vi "顶层容器-有线上位机.vi"() -> ()   [LabVIEW 2017]
panel:
  out "查-刷新设备表 按钮":refnum<vi>
  out "查-查询今日 按钮":refnum<vi>
  out "累积查询窗口VI-引用":refnum<vi>
  out "管-更新列表状态？":refnum<vi>
  out "管-停止信号（枚举）":refnum<vi>
  out "管-监测窗口 按钮":refnum<vi>
  in  "监-外部停止信号":refnum<vi>
  out "管理窗口VI-引用":refnum<vi>
  out "管-监测窗口VI-控件引用":refnum<vi>
  in  "管理模式":bool
  in  "监测模式":bool
  in  "累积查询":bool
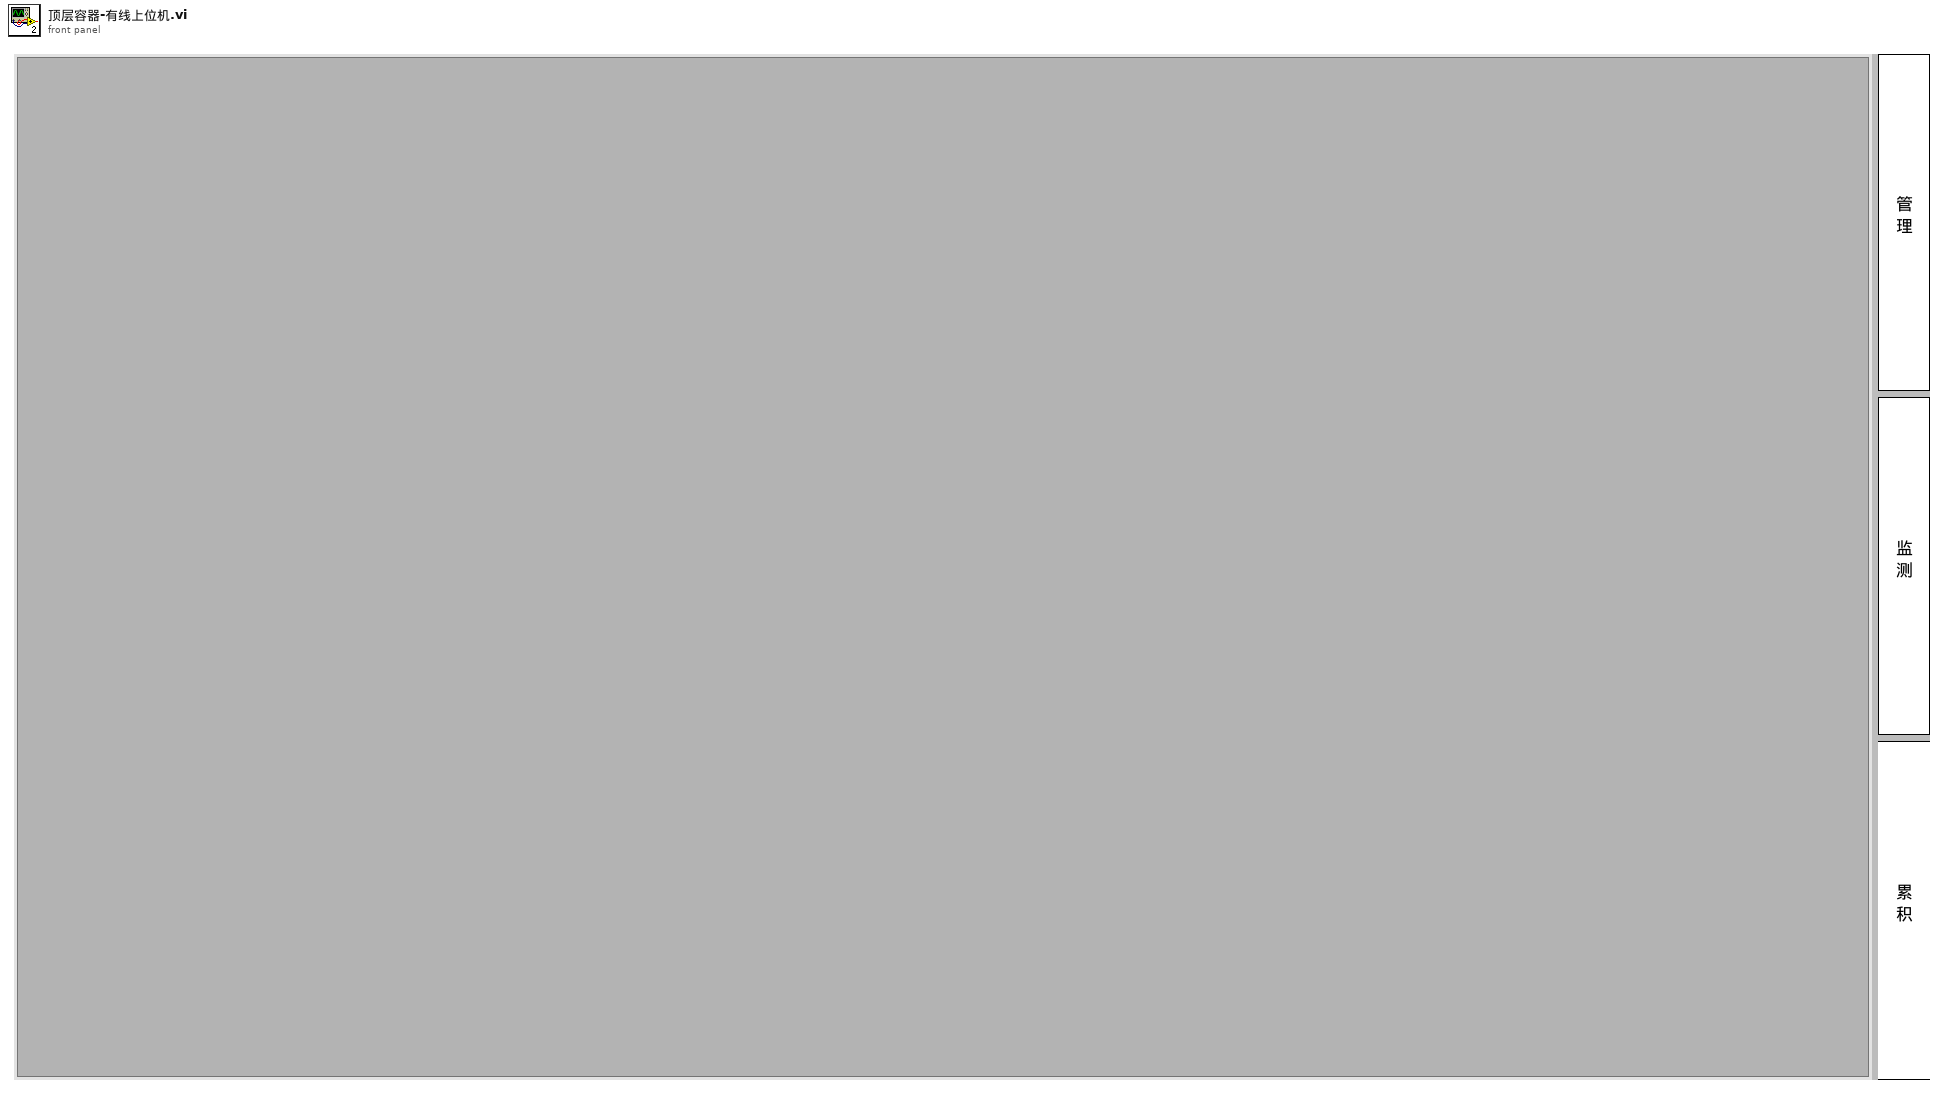
[diagram p1: front panel]
types:
  T1 = enum8{"Enabled", "Disabled", "Disabled and Grayed Out"}
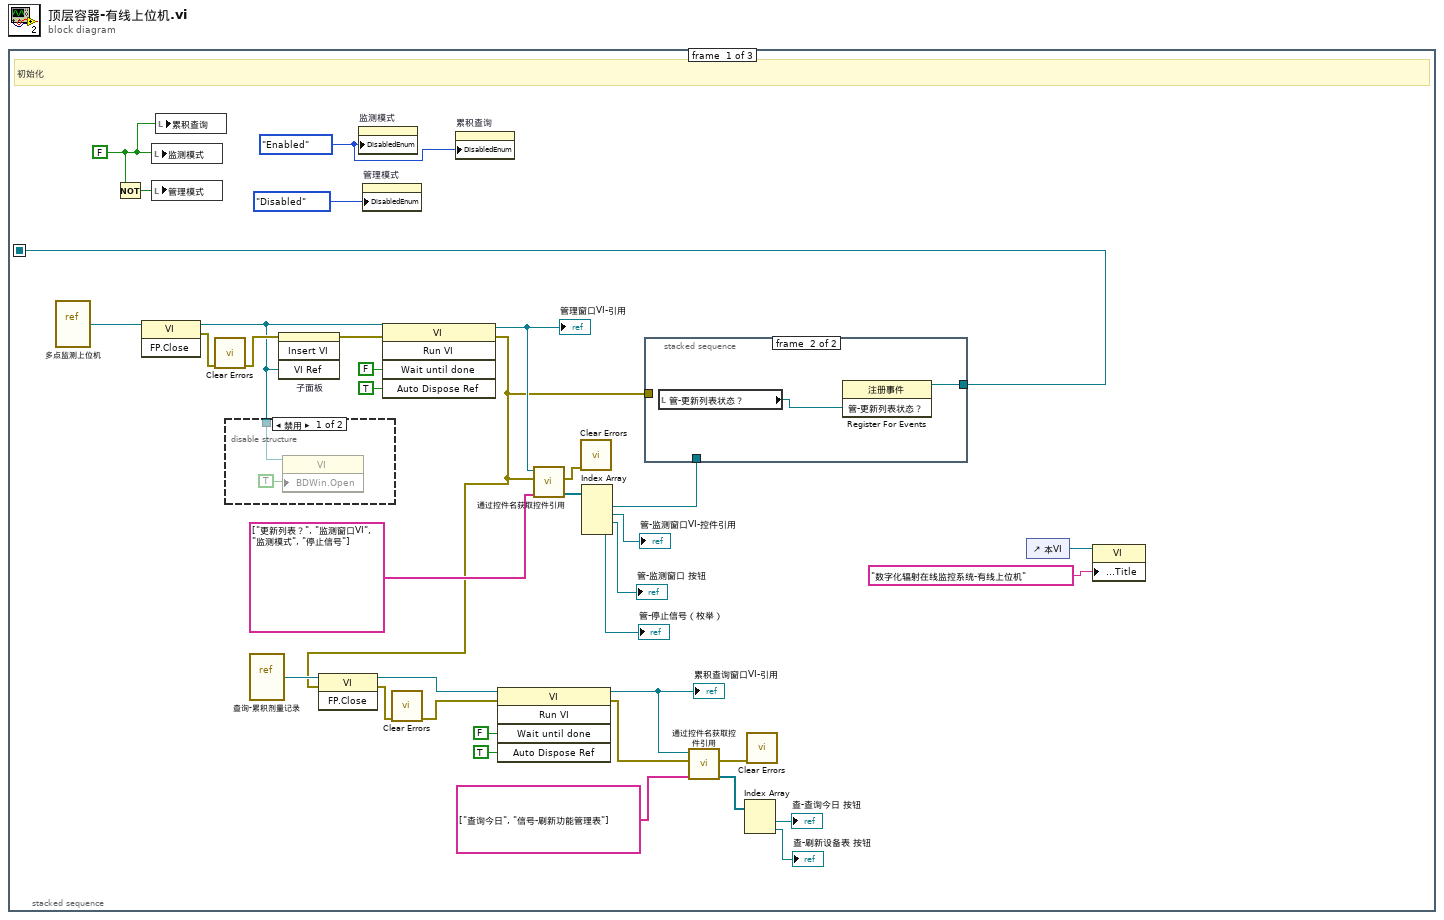
[diagram p0: block diagram]
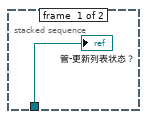
[diagram p3: hidden frame]
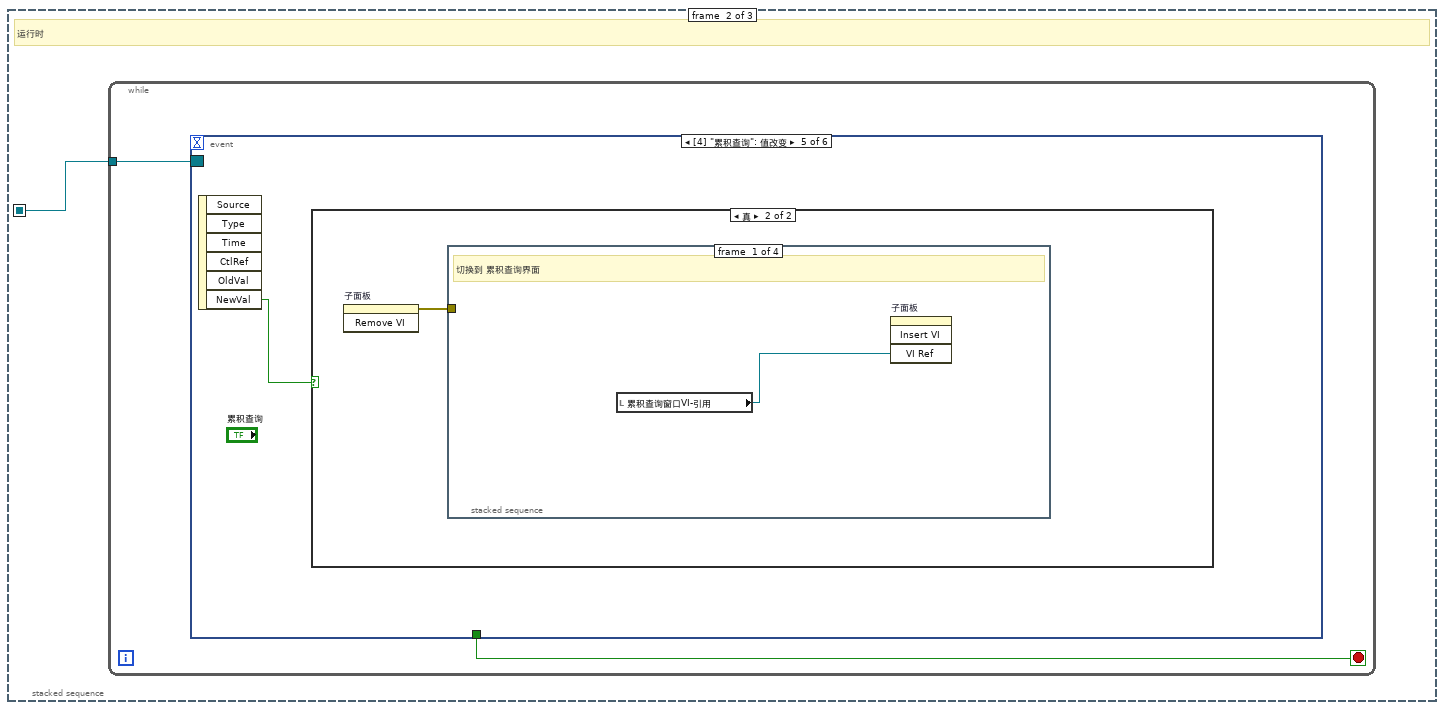
[diagram p4: hidden frame]
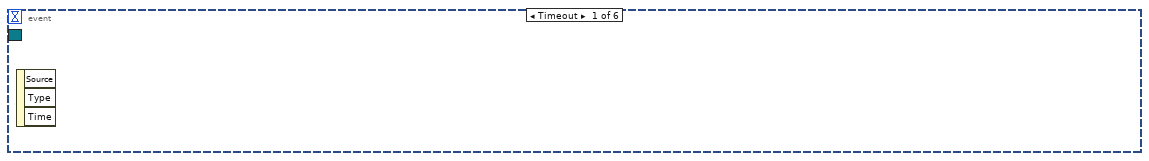
[diagram p5: hidden frame]
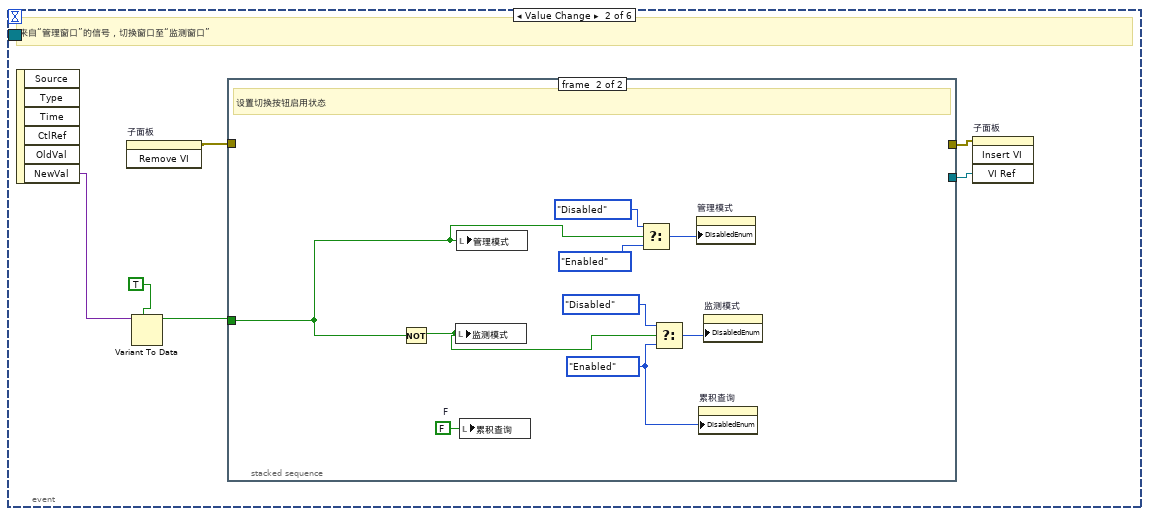
[diagram p6: hidden frame]
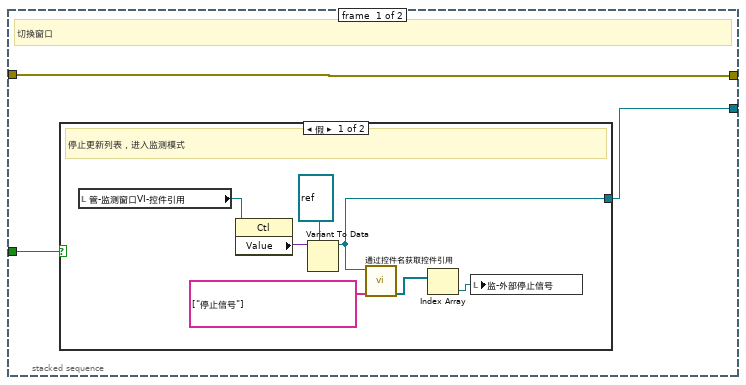
[diagram p7: hidden frame]
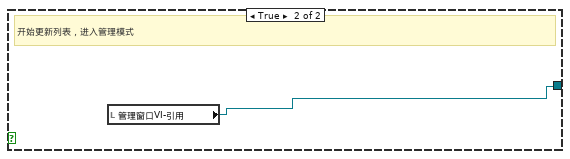
[diagram p8: hidden frame]
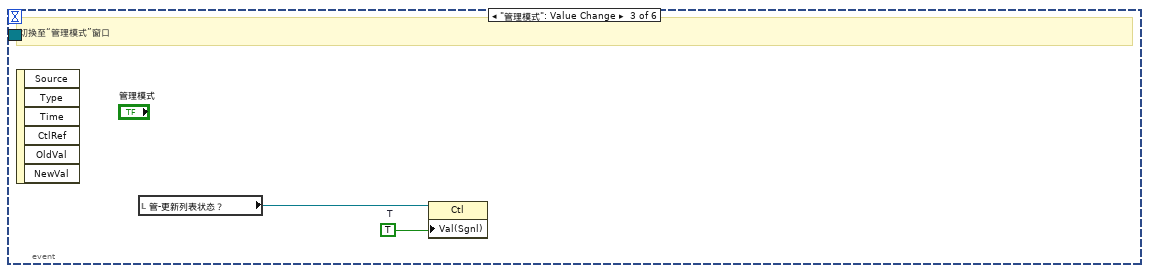
[diagram p9: hidden frame]
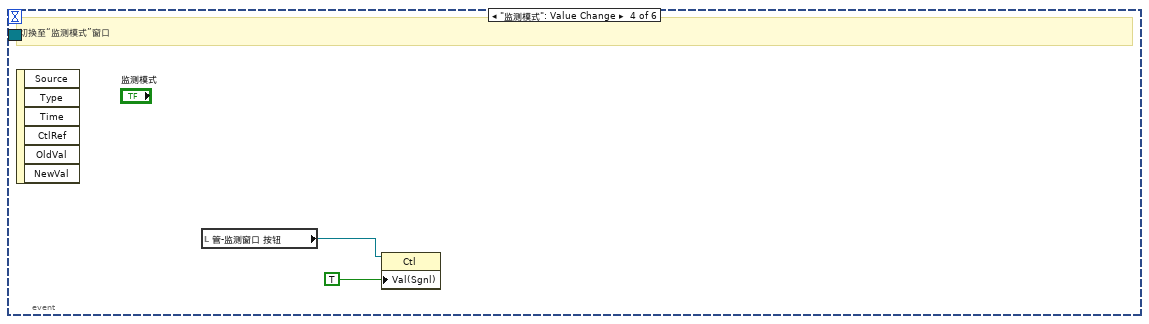
[diagram p10: hidden frame]
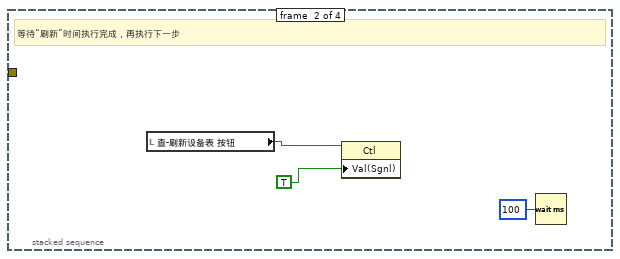
[diagram p12: hidden frame]
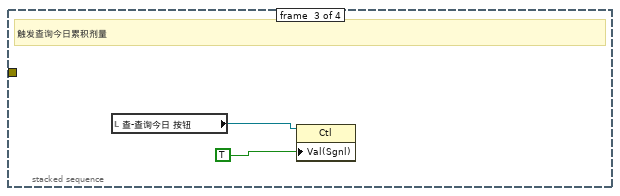
[diagram p13: hidden frame]
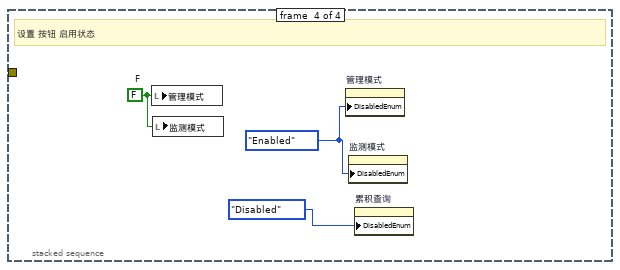
[diagram p14: hidden frame]
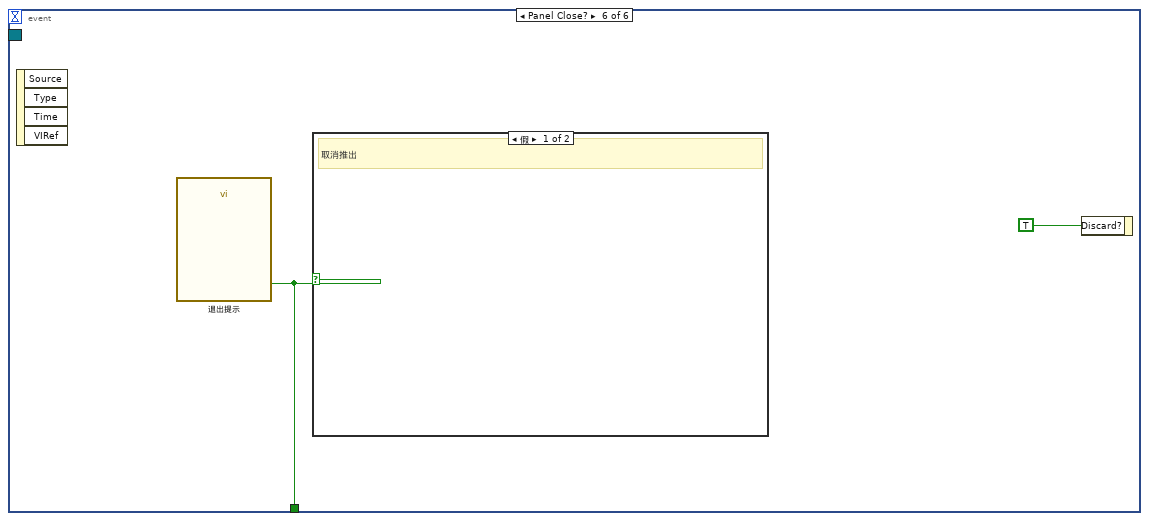
[diagram p15: hidden frame]
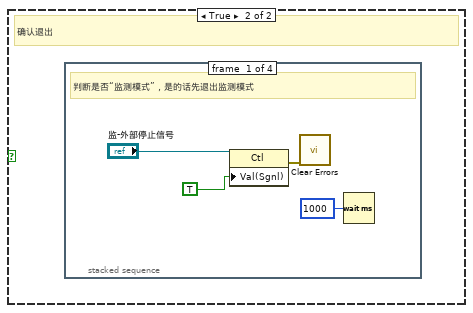
[diagram p16: hidden frame]
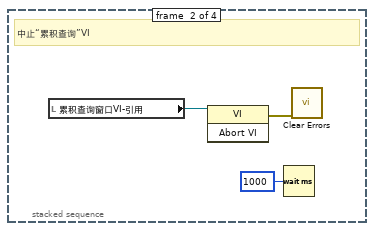
[diagram p17: hidden frame]
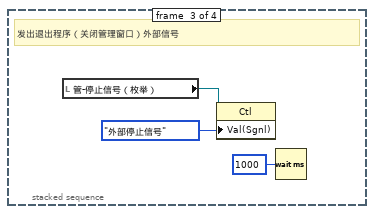
[diagram p18: hidden frame]
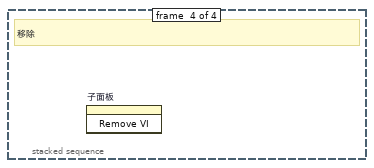
[diagram p19: hidden frame]
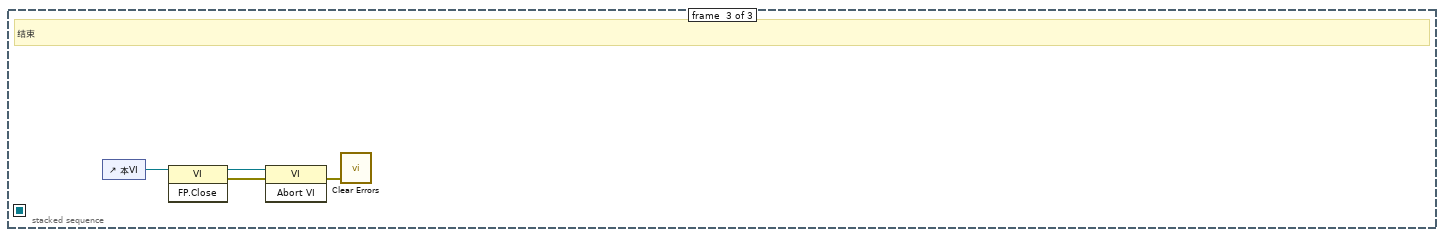
[diagram p20: hidden frame]
diagram:
  n1 = stacked-sequence {
    seq-local: [w31 _ _] -> [_ w42 _]
    frame #0 {
      w5 = T1."Enabled" ("禁用")
      w4 = FALSE ("监测模式")
      # "初始化"
      n2 = vi-ref "多点监测上位机.vi"() -> (w24:refnum<vi>)
      n3 = Not(x=w4) -> (.not. x?=w6:bool)
      n4 = invoke class="VI" method="FP.Close"(reference=w24) -> (reference out=w20:refnum<vi>, error out=w22:errorcluster)  [unwired: 2 in, 1 out]
      n5 = local write "监测模式"(w4) -> ()
      n6 = local write "管理模式"(w6) -> ()
      n7 = local write "累积查询"(w4) -> ()
      n8 = call <vilib>:"Clear Errors.vi"("error in (no error)"=w22) -> ("error out"=w21:errorcluster)  [unwired: 5 in, 1 out]
      n9 = disable-structure shown="禁用" {
        disable-tunnel: w20 -> [w38 _]
        frame Disabled {
          n10 = property class="VI"(reference=w38, "BDWin.Open"=TRUE ("程序框图窗口:打开")) -> ()  [unwired: 1 in, 2 out]
        }
        frame Enabled {
        }
      }
      n11 = vi-ref "查询-累积剂量记录.vi"() -> (w16:refnum<vi>)
      n12 = invoke on="子面板" class="子面板" method="Insert VI"(error in=w21, "VI Ref"=w20) -> (error out=w19:errorcluster)  [unwired: 2 in, 3 out]
      n13 = property on="监测模式" class="Bool (严格)"("DisabledEnum"=w5) -> ()  [unwired: 2 in, 2 out]
      n14 = property on="管理模式" class="Bool (严格)"("DisabledEnum"=T1."Disabled" ("禁用")) -> ()  [unwired: 2 in, 2 out]
      n15 = invoke class="VI" method="Run VI"(reference=w20, error in=w19, "Wait until done"=FALSE ("结束前等待"), "Auto Dispose Ref"=TRUE ("自动销毁引用")) -> (reference out=w32:refnum<vi>, error out=w1:errorcluster)  [unwired: 1 in, 3 out]
      "管理窗口VI-引用" <- w32
      n16 = invoke class="VI" method="FP.Close"(reference=w16, error in=w1) -> (reference out=w13:refnum<vi>, error out=w17:errorcluster)  [unwired: 1 in, 1 out]
      n17 = call <vilib>:"Clear Errors.vi"("error in (no error)"=w17) -> ("error out"=w12:errorcluster)  [unwired: 5 in, 1 out]
      n18 = property on="累积查询" class="Bool (严格)"("DisabledEnum"=w5) -> ()  [unwired: 2 in, 2 out]
      n19 = invoke class="VI" method="Run VI"(reference=w13, error in=w12, "Wait until done"=FALSE ("结束前等待"), "Auto Dispose Ref"=TRUE ("自动销毁引用")) -> (reference out=w2:refnum<vi>, error out=w9:errorcluster)  [unwired: 1 in, 3 out]
      "累积查询窗口VI-引用" <- w2
      n20 = call "通过控件名获取控件引用.vi"("控件名数组"=string[] ["更新列表？", "监测窗口VI", "监测模式", "停止信号"], "错误输入（无错误）"=w1, "VI引用"=w32) -> ("控件引用输出"=w34:refnum<vi>[], "错误输出"=w23:errorcluster)  [unwired: 6 in, 1 out]
      n21 = call <vilib>:"Clear Errors.vi"("error in (no error)"=w23) -> ()  [unwired: 5 in, 2 out]
      n22 = Index Array(array=w34) -> (element #1=w18:refnum<vi>, element #2=→"管-监测窗口VI-控件引用":refnum<vi>, element #3=→"管-监测窗口 按钮":refnum<vi>, element #4=→"管-停止信号（枚举）":refnum<vi>)  [unwired: 4 in]
      n23 = stacked-sequence {
        tunnel: [_ w41] -> w31
        tunnel: w1 -> [_ _]
        tunnel: w18 -> [w39 _]
        frame #0 {
          "管-更新列表状态？" <- w39
        }
        frame #1 {
          n24 = local read "管-更新列表状态？"() -> (w40:refnum<vi>)
          n25 = register-events(w40) -> (reference out=w41:refnum<event-registration>)  [unwired: 2 in, 1 out]
        }
      }
      n26 = call "通过控件名获取控件引用.vi"("控件名数组"=string[] ["查询今日", "信号-刷新功能管理表"], "错误输入（无错误）"=w9, "VI引用"=w2) -> ("控件引用输出"=w8:refnum<vi>[], "错误输出"=w11:errorcluster)  [unwired: 6 in, 1 out]
      n27 = Index Array(array=w8) -> (element #1=→"查-查询今日 按钮":refnum<vi>, element #2=→"查-刷新设备表 按钮":refnum<vi>)  [unwired: 2 in]
      n28 = call <vilib>:"Clear Errors.vi"("error in (no error)"=w11) -> ()  [unwired: 5 in, 2 out]
      n29 = control-ref of="本VI"() -> (w27:refnum<vi>)
      n30 = property class="VI"(reference=w27, "Front Panel.Title"="数字化辐射在线监控系统-有线上位机" ("前面板窗口:标题")) -> ()  [unwired: 1 in, 2 out]
    }
    frame #1 {
      # "运行时"
      n31 = while {
        tunnel: w42 -> [w43]
        stop <- w44 stop-if-true
        n32 = event shown="[4] \"累积查询\": 值改变" {
          selector: w43 -> [_ _ _ _ _ _]
          dyn-events: _ -> [_ _ _ _ _ _]
          timeout: _ -> [_ _ _ _ _ _]
          tunnel: [_ _ _ _ _ w86] -> w44
          event Timeout {
            n33 = event-data() -> ()  [unwired: 1 in, 3 out]
          }
          event Value Change {
            # "来自“管理窗口”的信号，切换窗口至“监测窗口”"
            n34 = event-data() -> ("NewVal"=w48:variant)  [unwired: 1 in, 5 out]
            n35 = invoke on="子面板" class="子面板" method="Remove VI"() -> (error out=w50:errorcluster)  [unwired: 3 in, 2 out]
            n36 = Variant To Data(type=TRUE, Variant=w48) -> (data=w47:bool)  [unwired: 1 in, 1 out]
            n37 = stacked-sequence {
              tunnel: w47 -> [w53 w67]
              tunnel: w50 -> [w51 _]
              tunnel: [w52 _] -> w45
              tunnel: [w51 _] -> w49
              frame #0 {
                # "切换窗口"
                n38 = case shown="假" w53 {
                  tunnel: [w54 w61] -> w52
                  frame False {
                    # "停止更新列表，进入监测模式"
                    n39 = local read "管-监测窗口VI-控件引用"() -> (w60:refnum<vi>)
                    n40 = property class="Ctl"(reference=w60) -> ("Value"=w59:variant)  [unwired: 1 in, 2 out]
                    n41 = Variant To Data(type=refnum<vi> refnum ("本VI"), Variant=w59) -> (data=w54:refnum<vi>)  [unwired: 1 in, 1 out]
                    n42 = call "通过控件名获取控件引用.vi"("控件名数组"=string[] ["停止信号"], "VI引用"=w54) -> ("控件引用输出"=w56:refnum<vi>[])  [unwired: 7 in, 2 out]
                    n43 = Index Array(array=w56) -> (element=w55:refnum<vi>)  [unwired: 1 in]
                    n44 = local write "监-外部停止信号"(w55) -> ()
                  }
                  frame True {
                    # "开始更新列表，进入管理模式"
                    n45 = local read "管理窗口VI-引用"() -> (w61:refnum<vi>)
                  }
                }
              }
              frame #1 {
                w63 = FALSE  # F
                w62 = T1."Enabled" ("禁用")
                # "设置切换按钮启用状态"
                n46 = Not(x=w67) -> (.not. x?=w64:bool)
                n47 = local write "监测模式"(w64) -> ()
                n48 = local write "管理模式"(w67) -> ()
                n49 = local write "累积查询"(w63) -> ()
                n50 = Select(t=T1."Disabled" ("禁用"), s=w67, f=T1."Enabled" ("禁用")) -> (s? t:f=w66:T1)
                n51 = Select(t=T1."Disabled" ("禁用"), s=w64, f=w62) -> (s? t:f=w65:T1)
                n52 = property on="管理模式" class="Bool (严格)"("DisabledEnum"=w66) -> ()  [unwired: 2 in, 2 out]
                n53 = property on="累积查询" class="Bool (严格)"("DisabledEnum"=w62) -> ()  [unwired: 2 in, 2 out]
                n54 = property on="监测模式" class="Bool (严格)"("DisabledEnum"=w65) -> ()  [unwired: 2 in, 2 out]
              }
            }
            n55 = invoke on="子面板" class="子面板" method="Insert VI"(error in=w49, "VI Ref"=w45) -> ()  [unwired: 2 in, 4 out]
          }
          event "管理模式": Value Change {
            w72 = TRUE  # T
            # "切换至“管理模式”窗口"
            n56 = event-data() -> ()  [unwired: 1 in, 6 out]
            n57 = local read "管-更新列表状态？"() -> (w71:refnum<vi>)
            n58 = property class="Ctl"(reference=w71, "Val(Sgnl)"=w72) -> ()  [unwired: 1 in, 2 out]
          }
          event "监测模式": Value Change {
            # "切换至“监测模式”窗口"
            n59 = event-data() -> ()  [unwired: 1 in, 6 out]
            n60 = local read "管-监测窗口 按钮"() -> (w74:refnum<vi>)
            n61 = property class="Ctl"(reference=w74, "Val(Sgnl)"=TRUE ("监测模式")) -> ()  [unwired: 1 in, 2 out]
          }
          event "累积查询": Value Change {
            n62 = event-data() -> ("NewVal"=w75:bool)  [unwired: 1 in, 5 out]
            n63 = case shown="真" w75 {
              frame False {
              }
              frame True {
                n64 = invoke on="子面板" class="子面板" method="Remove VI"() -> (error out=w76:errorcluster)  [unwired: 3 in, 2 out]
                n65 = stacked-sequence {
                  tunnel: w76 -> [_ _ _ _]
                  frame #0 {
                    # "切换到 累积查询界面"
                    n66 = local read "累积查询窗口VI-引用"() -> (w77:refnum<vi>)
                    n67 = invoke on="子面板" class="子面板" method="Insert VI"("VI Ref"=w77) -> ()  [unwired: 3 in, 4 out]
                  }
                  frame #1 {
                    # "等待“刷新”时间执行完成，再执行下一步"
                    n68 = local read "查-刷新设备表 按钮"() -> (w80:refnum<vi>)
                    n69 = property class="Ctl"(reference=w80, "Val(Sgnl)"=TRUE) -> ()  [unwired: 1 in, 2 out]
                    n70 = Wait (ms)(milliseconds to wait=u32 100 ("等待时间（毫秒）")) -> ()  [unwired: 1 out]
                  }
                  frame #2 {
                    # "触发查询今日累积剂量"
                    n71 = local read "查-查询今日 按钮"() -> (w82:refnum<vi>)
                    n72 = property class="Ctl"(reference=w82, "Val(Sgnl)"=TRUE) -> ()  [unwired: 1 in, 2 out]
                  }
                  frame #3 {
                    w85 = FALSE  # F
                    w83 = T1."Enabled" ("禁用")
                    # "设置 按钮 启用状态"
                    n73 = local write "管理模式"(w85) -> ()
                    n74 = local write "监测模式"(w85) -> ()
                    n75 = property on="管理模式" class="Bool (严格)"("DisabledEnum"=w83) -> ()  [unwired: 2 in, 2 out]
                    n76 = property on="监测模式" class="Bool (严格)"("DisabledEnum"=w83) -> ()  [unwired: 2 in, 2 out]
                    n77 = property on="累积查询" class="Bool (严格)"("DisabledEnum"=T1."Disabled" ("禁用")) -> ()  [unwired: 2 in, 2 out]
                  }
                }
              }
            }
          }
          event Panel Close? {
            n78 = event-data() -> ()  [unwired: 1 in, 4 out]
            n79 = call "退出提示"() -> ("确定"=w86:bool)  [unwired: 10 in, 1 out]
            n80 = case shown="假" w86 {
              frame False {
                # "取消推出"
              }
              frame True {
                # "确认退出"
                n81 = stacked-sequence {
                  frame #0 {
                    # "判断是否“监测模式”，是的话先退出监测模式"
                    n82 = property class="Ctl"(reference="监-外部停止信号", "Val(Sgnl)"=TRUE ("监测模式")) -> (error out=w90:errorcluster)  [unwired: 1 in, 1 out]
                    n83 = call <vilib>:"Clear Errors.vi"("error in (no error)"=w90) -> ()  [unwired: 5 in, 2 out]
                    n84 = Wait (ms)(milliseconds to wait=u32 1000 ("等待时间（毫秒）")) -> ()  [unwired: 1 out]
                  }
                  frame #1 {
                    # "中止“累积查询”VI"
                    n85 = local read "累积查询窗口VI-引用"() -> (w94:refnum<vi>)
                    n86 = invoke class="VI" method="Abort VI"(reference=w94) -> (error out=w92:errorcluster)  [unwired: 2 in, 2 out]
                    n87 = Wait (ms)(milliseconds to wait=u32 1000 ("等待时间（毫秒）")) -> ()  [unwired: 1 out]
                    n88 = call <vilib>:"Clear Errors.vi"("error in (no error)"=w92) -> ()  [unwired: 5 in, 2 out]
                  }
                  frame #2 {
                    # "发出退出程序（关闭管理窗口）外部信号"
                    n89 = local read "管-停止信号（枚举）"() -> (w97:refnum<vi>)
                    n90 = property class="Ctl"(reference=w97, "Val(Sgnl)"=enum16{"内部停止信号", "外部停止信号"}."外部停止信号" ("值(信号)")) -> ()  [unwired: 1 in, 2 out]
                    n91 = Wait (ms)(milliseconds to wait=u32 1000 ("等待时间（毫秒）")) -> ()  [unwired: 1 out]
                  }
                  frame #3 {
                    # "移除"
                    n92 = invoke on="子面板" class="子面板" method="Remove VI"() -> ()  [unwired: 3 in, 3 out]
                  }
                }
              }
            }
            n93 = event-data("Discard?"=TRUE ("放弃？")) -> ()  [unwired: 1 in, 1 out]
          }
        }
      }
    }
    frame #2 {
      # "结束"
      n94 = control-ref of="本VI"() -> (w101:refnum<vi>)
      n95 = invoke class="VI" method="FP.Close"(reference=w101) -> (reference out=w100:refnum<vi>, error out=w99:errorcluster)  [unwired: 2 in, 1 out]
      n96 = invoke class="VI" method="Abort VI"(reference=w100, error in=w99) -> (error out=w98:errorcluster)  [unwired: 1 in, 2 out]
      n97 = call <vilib>:"Clear Errors.vi"("error in (no error)"=w98) -> ()  [unwired: 5 in, 2 out]
    }
  }
